vi "testCamera3.vi"() -> ()   [LabVIEW 2018]
uses:
  <vilib>/userdefined/High Color/IMAQdx.ctl
  vision/vision info 2.vi
  <vilib>/vision/driver/NI_Vision_Acquisition_Software.lvlib
  <resource>/objmgr/imaqdx.rc
panel:
  out "Image 2":T1(plugin-control)
  out "Circles":cluster{"x":dbl, "y":dbl, "r":dbl}[](array[cluster])
  out "Circles 2":cluster{"x":dbl, "y":dbl, "r":dbl}[](array[cluster])
  out "size(s)":i32
  out "Image":T1(plugin-control)
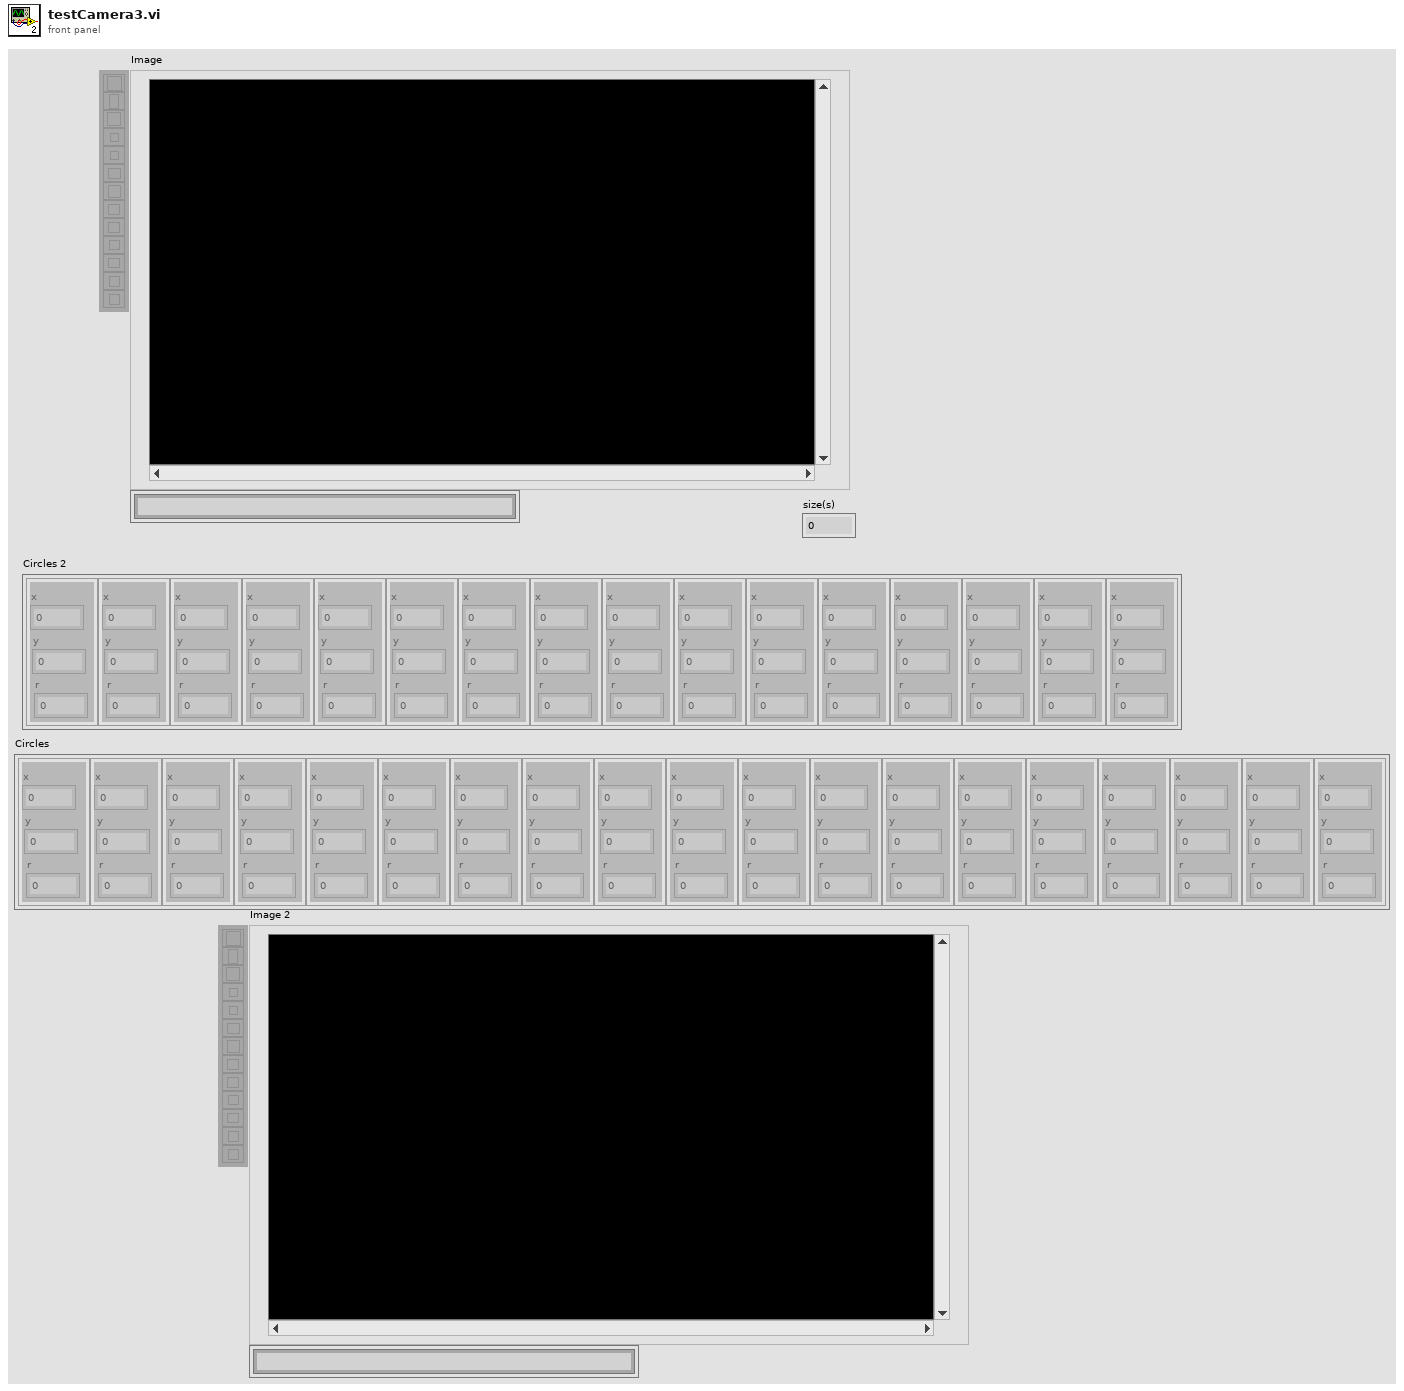
[diagram p1: front panel]
types:
  T1 = typedef "IMAQ Image.ctl" = refnum<image>
  T2 = typedef "IMAQdx.ctl" = refnum<k21>
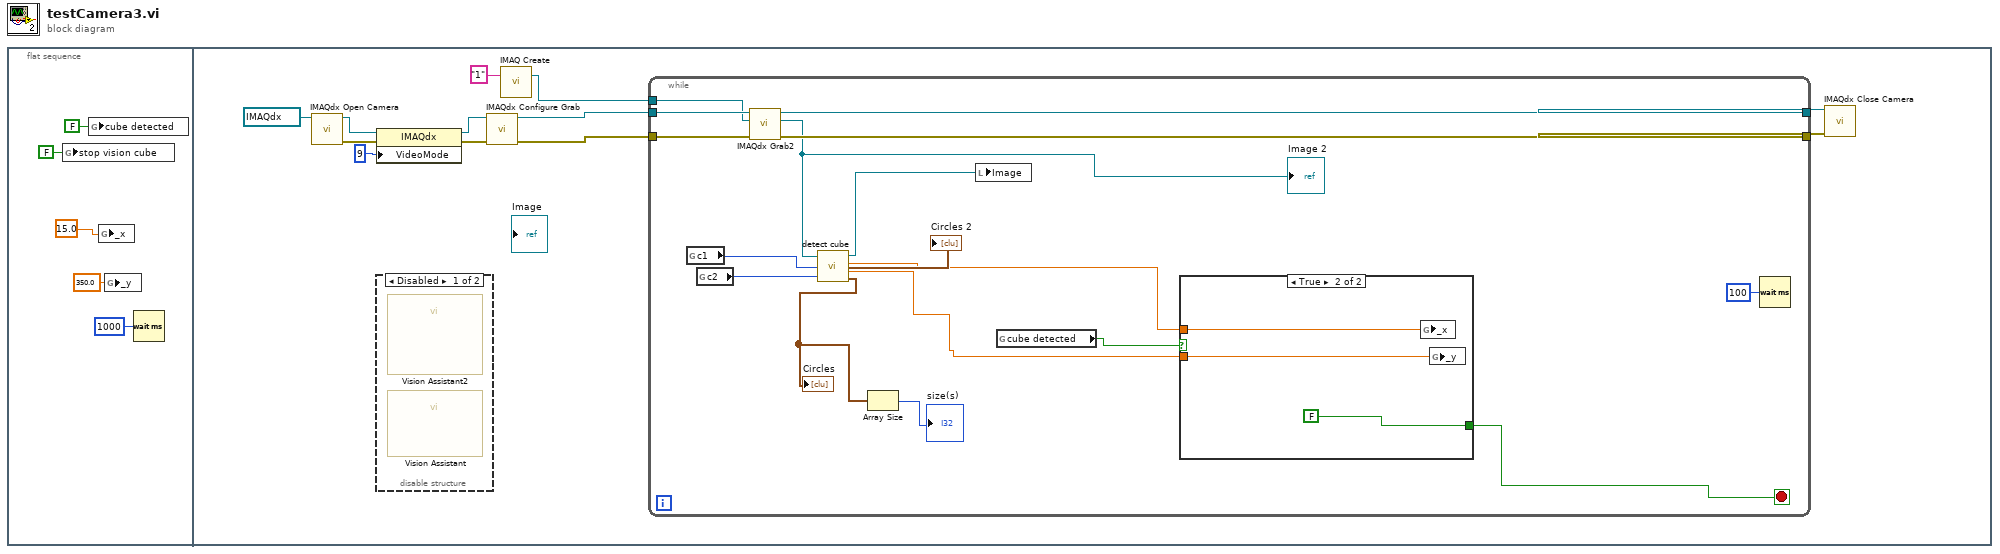
[diagram p0: block diagram]
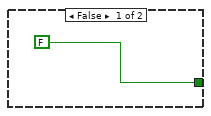
[diagram p3: hidden frame]
diagram:
  n1 = flat-sequence {
    frame #0 {
      n2 = global write "vision info 2.vi" "stop vision cube"(FALSE ("stop vision cube")) -> ()
      n3 = global write "vision info 2.vi" "cube detected"(FALSE ("cube detected")) -> ()
      n4 = global write "vision info 2.vi" "_x"(15.0 ("_x")) -> ()
      n5 = global write "vision info 2.vi" "_y"(350.0 ("_y")) -> ()
      n6 = Wait (ms)(milliseconds to wait=u32 1000) -> ()  [unwired: 1 out]
    }
    frame #1 {
      n7 = call <vilib>:"IMAQdx Open Camera.vi"("Session In"=T2 "cam2") -> ("error out"=w9:errorcluster, "Session Out"=w10:T2)  [unwired: 9 in]
      n8 = property class="IMAQdx"(reference=w10, error in=w9, "VideoMode"=u32 9) -> (reference out=w7:T2, error out=w8:errorcluster)
      n9 = disable-structure shown="Disabled" {
        frame Disabled {
          n10 = call "Vision Assistant2"() -> ()  [unwired: 26 in, 2 out]
          n11 = call "Vision Assistant"() -> ()  [unwired: 26 in, 2 out]
        }
        frame Enabled {
        }
      }
      n12 = call <vilib>:"IMAQdx Configure Grab.vi"("error in"=w8, "Session In"=w7) -> ("error out"=w16:errorcluster, "Session Out"=w15:T2)  [unwired: 8 in]
      n13 = call "IMAQ Create"("Image Name"="1") -> ("New Image"=w13:T1)  [unwired: 4 in, 1 out]
      n14 = while {
        tunnel: w16 -> [w34]
        tunnel: w15 -> [w33]
        tunnel: [w32] -> w14
        tunnel: w13 -> [w31]
        tunnel: [w30] -> w11
        stop <- w28 stop-if-true
        n15 = global read "vision info 2.vi" "c1"() -> (w25:i8)
        n16 = global read "vision info 2.vi" "c2"() -> (w24:i8)
        n17 = call <vilib>:"IMAQdx Grab2.vi"("error in"=w34, "Image In"=w31, "Session In"=w33) -> ("error out"=w30:errorcluster, "Image Out"=w26:T1, "Session Out"=w32:T2)  [unwired: 5 in, 1 out]
        "Image 2" <- w26
        n18 = call "detect cube.vi"("Image 3"=w26, "c1"=w25, "c2"=w24) -> ("Image 4"=w27:T1, "_x"=w21:dbl, "_y"=w20:dbl, "Circles"=w23:cluster{"x":dbl, "y":dbl, "r":dbl}[], "Circles 2"=→"Circles 2":cluster{"x":dbl, "y":dbl, "r":dbl}[])
        "Circles" <- w23
        n19 = Array Size(array=w23) -> (size(s)=→"size(s)":i32)
        n20 = local write "Image"(w27) -> ()
        n21 = global read "vision info 2.vi" "cube detected"() -> (w18:bool)
        n22 = case shown="True" w18 {
          tunnel: w21 -> [_ w38]
          tunnel: w20 -> [_ w37]
          tunnel: [FALSE ("stop vision cube") FALSE ("stop vision cube")] -> w28
          frame False {
          }
          frame True {
            n23 = global write "vision info 2.vi" "_x"(w38) -> ()
            n24 = global write "vision info 2.vi" "_y"(w37) -> ()
          }
        }
        n25 = Wait (ms)(milliseconds to wait=u32 100) -> ()  [unwired: 1 out]
      }
      n26 = call <vilib>:"IMAQdx Close Camera.vi"("error in"=w11, "Session In"=w14) -> ()  [unwired: 9 in, 1 out]
    }
  }
